vi "Lissajous Round.vi"() -> ()   [LabVIEW 2020]
panel:
  out "XY Graph":cluster{dbl, dbl}[](graph)
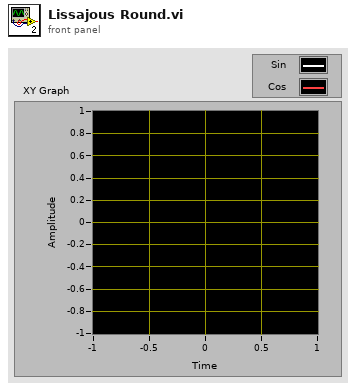
[diagram p1: front panel]
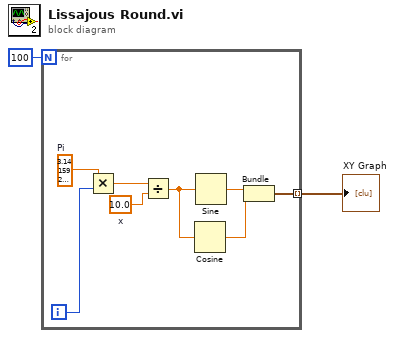
[diagram p0: block diagram]
diagram:
  n1 = for {
    N: 100 -> [_]
    tunnel: [w3] -> w1 mode=indexing
    i -> [w10]
    w7 = 10.0  # x
    w9 = 3.141592653589793  # Pi
    n2 = Multiply(x=w9, y=w10) -> (x*y=w8:dbl)
    n3 = Divide(x=w8, y=w7) -> (x/y=w6:dbl)
    n4 = Cosine(x=w6) -> (cos(x)=w4:dbl)
    n5 = Sine(x=w6) -> (sin(x)=w5:dbl)
    n6 = Bundle(w5, w4) -> (w3:cluster{dbl, dbl})  [unwired: 1 in]
  }
  "XY Graph" <- w1
